vi "crop_input_images_float.vi"() -> ()   [LabVIEW 2011]
uses:
  global_vars.vi
  <vilib>/Utility/file.llb/Write To Spreadsheet File (I64).vi
panel:
  in  "dbl_gamma_correction":dbl=1.0
  in  "dbl_noise_threshold":dbl=20.0
  in  "update global variables":bool
  out "i32_First/last px":i32[][](graph)
  in  "safety margin":i32=5
  out "u8_ar_noise_mask":u8[][](array[numeric])
  out "input_line_plot 2":dbl[][](graph)
  in  "Tab Control":T1(tab)
  out "input_line_plot":dbl[][](graph)
  out "img_dist_input":T2(plugin-control)
  out "img_orig_input":T2(plugin-control)
  in  "i32_sel_input_image":i32
  in  "select row input":i32(slide) scale=0.0..1200.0
  in  "select row unwrapped":i32(slide) scale=0.0..1200.0
  out "img_dist_phaseMap":T2(plugin-control)
  out "img_orig_masked_with_dist":T2(plugin-control)
  out "noise_mask_line_plot":i32[](graph)
  in  "select row":i32(slide) scale=0.0..1200.0
  out "last px":i32
  out "first px":i32
  out "img_noise_mask":T2(plugin-control)
  in  "save data":bool
  out "i32_ar_displ_map":i32[][](array[numeric])
  out "crunching numbers":bool
  out "Intensity Graph":i32[][](graph)
  out "img_orig_unwrap":T2(plugin-control)
  in  "calc difference":bool
  out "Y Resolution":i32
  out "X Resolution":i32
  in  "update_cor":bool
  out "path_dist_files":path[](array[path])=[path "X:/Cloud Drives/Dropbox/Europhotonics/FringeMan/Image Storage/02_07/x-direction/dist/12_56_10-5.00fringes_0of4__capt_.png", path "X:/Cloud Drives/Dropbox/Europhotonics/FringeMan/Image Storage/02_07/x-direction/dist/12_56_10-5.00fringes_1of4__capt_.png", path "X:/Cloud Drives/Dropbox/Europhotonics/FringeMan/Image Storage/02_07/x-direction/dist/12_56_10-5.00fringes_2of4__capt_.png", path "X:/Cloud Drives/Dropbox/Europhotonics/FringeMan/Image Storage/02_07/x-direction/dist/12_56_10-5.00fringes_3of4__capt_.png"]
  out "path_orig_files":path[](array[path])=[path "X:/Cloud Drives/Dropbox/Europhotonics/FringeMan/Image Storage/02_07/x-direction/orig/12_56_10-5.00fringes_0of4__original_.png", path "X:/Cloud Drives/Dropbox/Europhotonics/FringeMan/Image Storage/02_07/x-direction/orig/12_56_10-5.00fringes_1of4__original_.png", path "X:/Cloud Drives/Dropbox/Europhotonics/FringeMan/Image Storage/02_07/x-direction/orig/12_56_10-5.00fringes_2of4__original_.png", path "X:/Cloud Drives/Dropbox/Europhotonics/FringeMan/Image Storage/02_07/x-direction/orig/12_56_10-5.00fringes_3of4__original_.png"]
  in  "dbl_ar_crop_correction":dbl[](array[numeric])=[0.0, 0.0, 0.0, 0.0] caption="crop_correction"
  in  "u8_y_center_cor":i16
  in  "u8_x_center_cor":i16=-20
  in  "radius correction":i16=-30
  out "img_dist_unwrap":T2(plugin-control)
  out "u8_ar_orig_phasemap":dbl[][](array[numeric])
  out "dbl_pxar_orig_unwrap":dbl[][](array[numeric])
  out "dbl_pxar_dist_unwrap":dbl[][](array[numeric])
  out "u8_pxar_orig":dbl[][][](array[numeric])
  in  "read orig":bool
  in  "read dist":bool
  out "u8_ar_dist_phasemap":dbl[][](array[numeric])
  in  "calculate \nphase map":bool
  out "u8_pxar_dist":dbl[][][](array[numeric])
  in  "Stop Button":bool
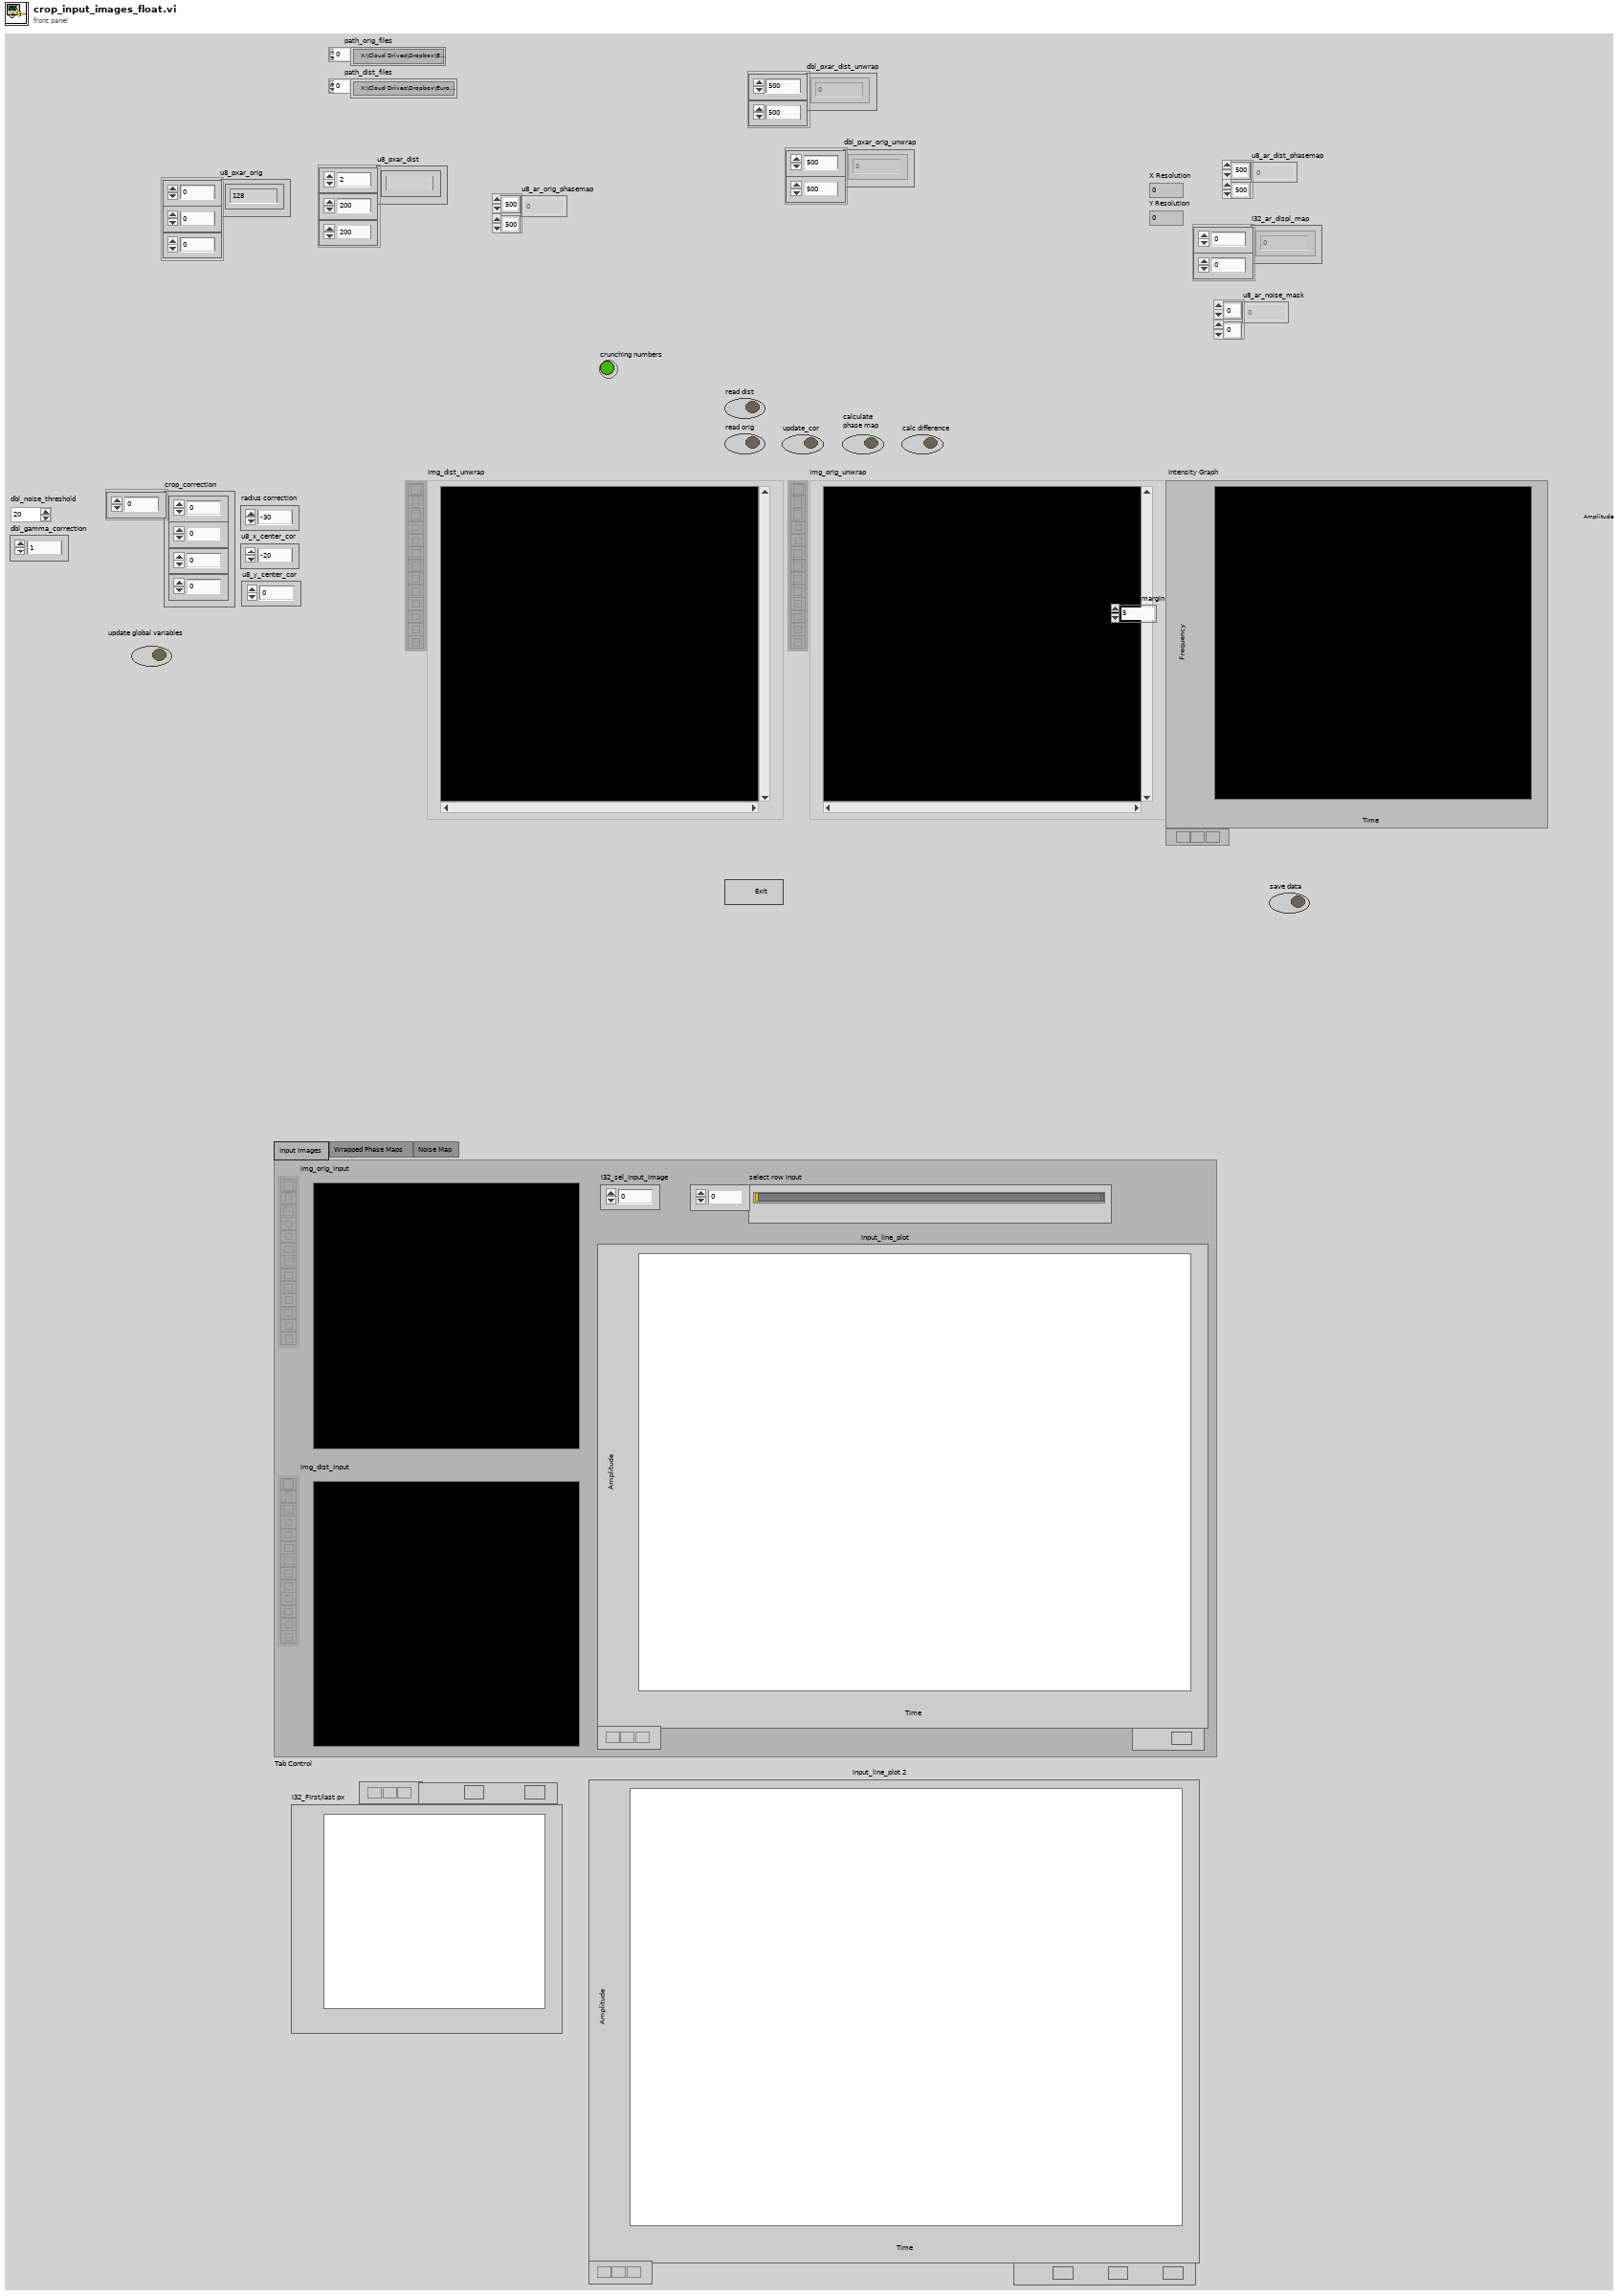
[diagram p1: front panel]
types:
  T1 = enum32{"Input Images", "Wrapped Phase Maps", "Noise Map"}
  T2 = typedef "IMAQ Image.ctl" = refnum<image>
  T3 = cluster{"radius correction":i16, "u8_x_center_cor":i16, "u8_y_center_cor":i16}
  T4 = typedef "Image Type" = u32
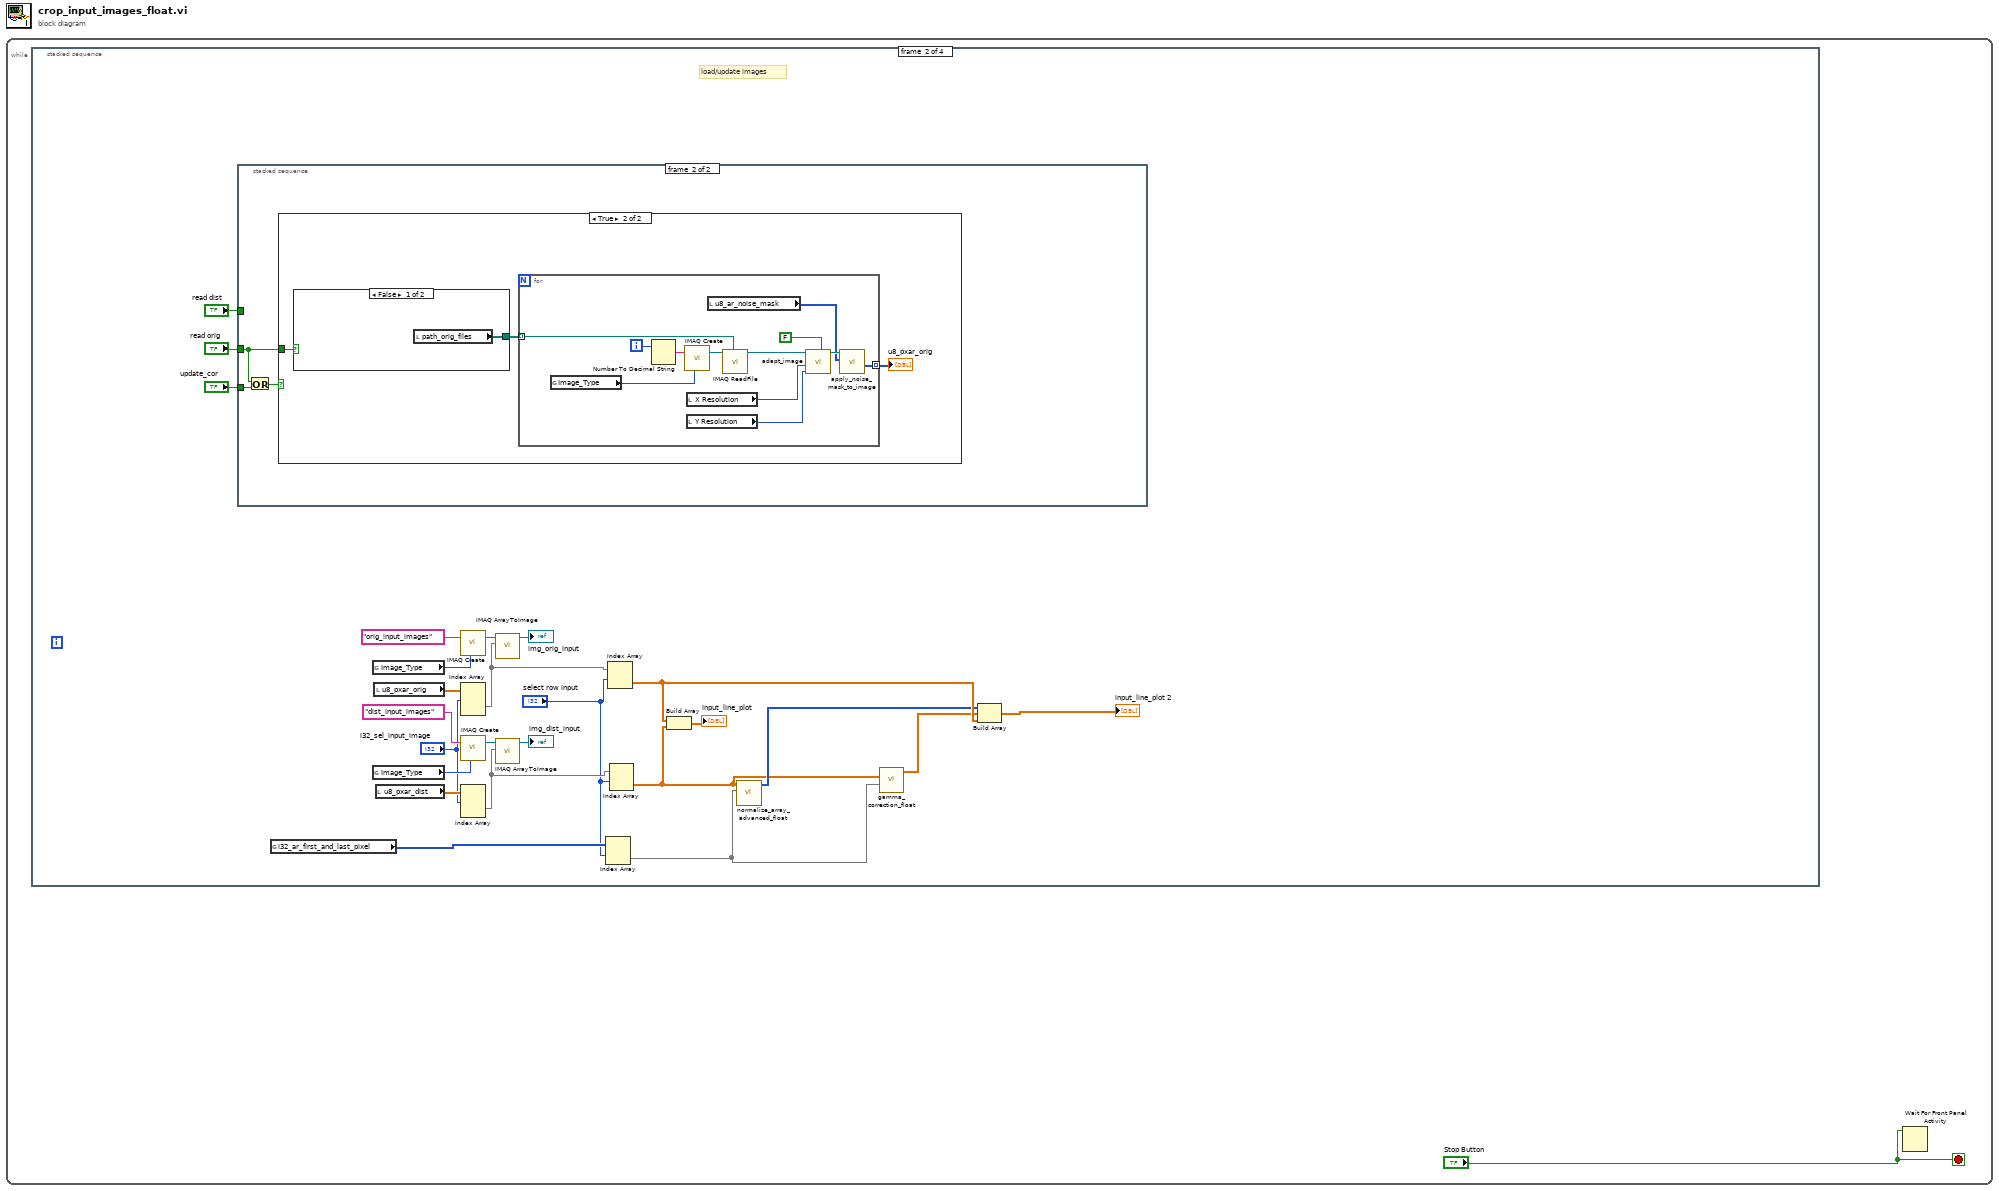
[diagram p0: block diagram]
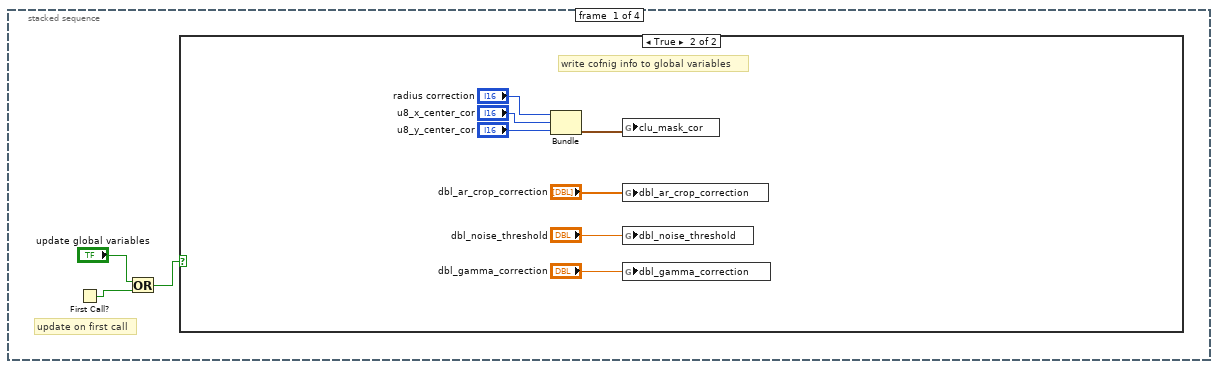
[diagram p2: hidden frame]
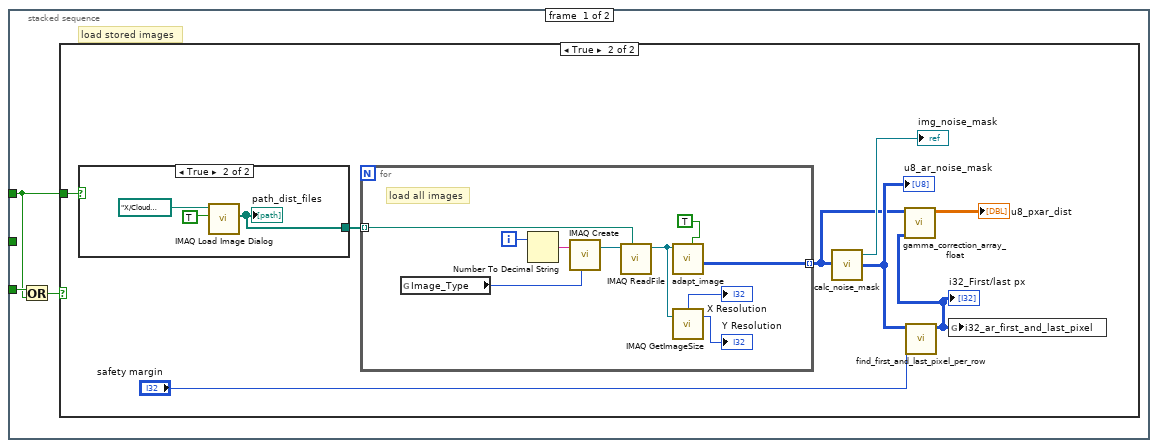
[diagram p4: hidden frame]
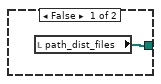
[diagram p6: hidden frame]
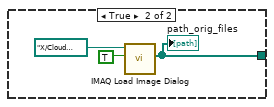
[diagram p8: hidden frame]
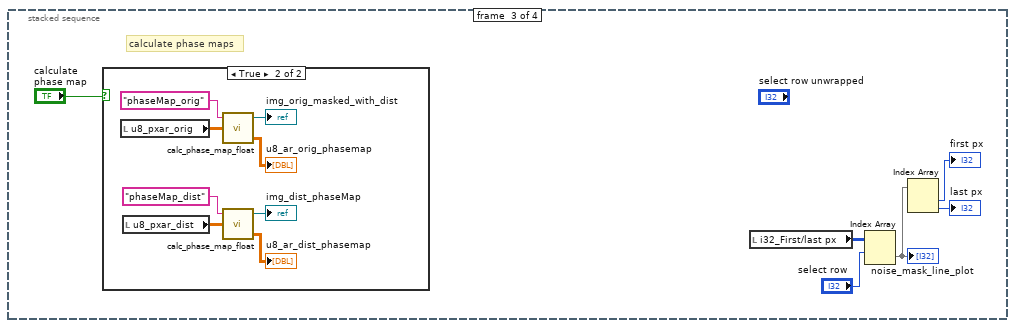
[diagram p9: hidden frame]
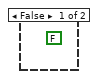
[diagram p10: hidden frame]
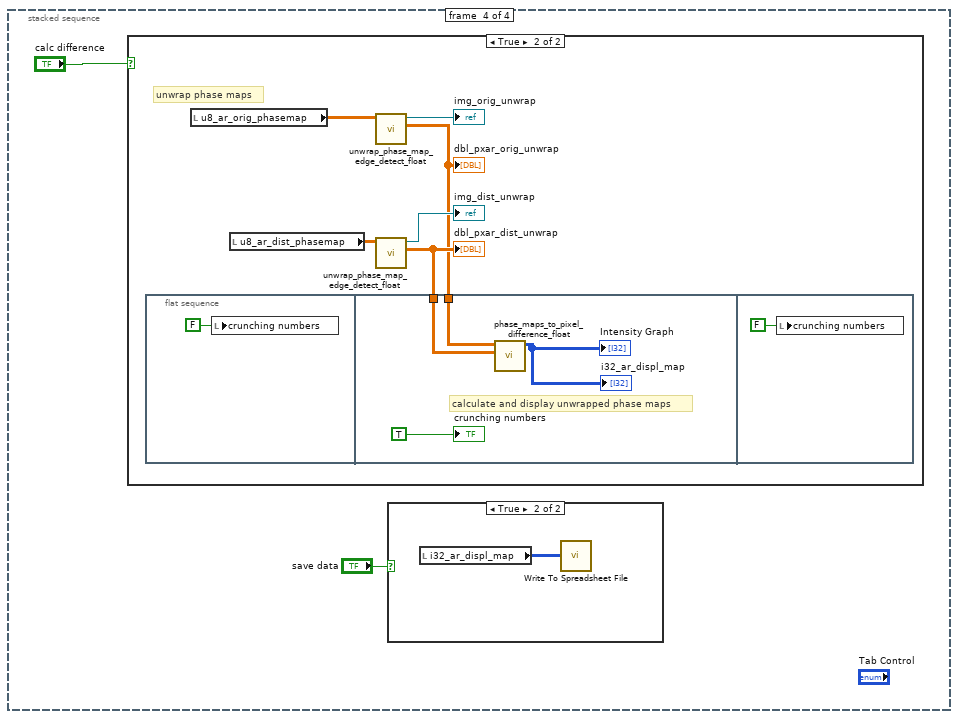
[diagram p11: hidden frame]
diagram:
  n1 = while {
    stop <- "Stop Button" stop-if-true
    n2 = stacked-sequence {
      frame #0 {
        # "update on first call"
        n3 = First Call?() -> (First Call?: T/F=w2:bool)
        n4 = Or(x="update global variables", y=w2) -> (x .or. y?=w3:bool)
        n5 = case shown="True" w3 {
          frame False {
          }
          frame True {
            # "write cofnig info to global variables"
            n6 = Bundle("radius correction"="radius correction", "u8_x_center_cor"="u8_x_center_cor", "u8_y_center_cor"="u8_y_center_cor") -> (w11:T3)  [unwired: 1 in]
            n7 = global write "global_vars.vi" "clu_mask_cor"(w11) -> ()
            n8 = global write "global_vars.vi" "dbl_ar_crop_correction"("dbl_ar_crop_correction") -> ()
            n9 = global write "global_vars.vi" "dbl_noise_threshold"("dbl_noise_threshold") -> ()
            n10 = global write "global_vars.vi" "dbl_gamma_correction"("dbl_gamma_correction") -> ()
          }
        }
      }
      frame #1 {
        # "load/update images"
        n11 = stacked-sequence {
          tunnel: "update_cor" -> [w39 w63]
          tunnel: "read dist" -> [w37 _]
          tunnel: "read orig" -> [_ w62]
          frame #0 {
            # "load stored images"
            n12 = Or(x=w39, y=w37) -> (x .or. y?=w38:bool)
            n13 = case shown="True" w38 {
              tunnel: w37 -> [_ w46]
              frame False {
              }
              frame True {
                n14 = case shown="True" w46 {
                  tunnel: [w48 w51] -> w47
                  frame False {
                    n15 = local read "path_dist_files"() -> (w48:path[])
                  }
                  frame True {
                    n16 = call "IMAQ Load Image Dialog"("Multiple Files? (No)"=TRUE, "Start Path"=path "X:/Cloud Drives/Dropbox/Europhotonics/FringeMan/Image Storage") -> ("Paths"=w51:path[])  [unwired: 7 in, 2 out]
                    "path_dist_files" <- w51
                  }
                }
                n17 = for {
                  tunnel: w47 -> [w57] mode=indexing
                  tunnel: [w53] -> w42 mode=indexing
                  i -> [w61]
                  # "load all images"
                  n18 = global read "global_vars.vi" "Image_Type"() -> (w58:T4)
                  n19 = Number To Decimal String(number=w61) -> (decimal integer string=w60:string)  [unwired: 1 in]
                  n20 = call "IMAQ Create"("Image Name"=w60, "Image Type"=w58) -> ("New Image"=w59:T2)  [unwired: 2 in, 2 out]
                  n21 = call "IMAQ ReadFile"("File Path"=w57, "Image"=w59) -> ("Image Out"=w54:T2)  [unwired: 5 in, 4 out]
                  n22 = call "adapt_image.vi"("captured image?"=TRUE, "orig_imageIn"=w54) -> ("adapted image px array"=w53:u8[][])  [unwired: 7 in, 2 out]
                  n23 = call "IMAQ GetImageSize"("Image"=w54) -> ("Y Resolution"=→"Y Resolution":i32, "X Resolution"=→"X Resolution":i32)  [unwired: 3 in, 1 out]
                }
                n24 = call "calc_noise_mask.vi"("u8_ar_image_pixel_array"=w42) -> ("u8_ar_noise_mask"=w43:u8[][], "img_noise mask"=→"img_noise_mask":T2)  [unwired: 3 in]
                "u8_ar_noise_mask" <- w43
                n25 = call "find_first_and_last_pixel_per_row.vi"("safety margin"="safety margin", "u8_ar_mask"=w43) -> ("i32_ar_first_and_last_pixel"=w40:i32[][])  [unwired: 9 in]
                "i32_First/last px" <- w40
                n26 = call "gamma_correction_array_float.vi"("i32_ar_first_and_last_pixel"=w40, "adapted image px array"=w42) -> ("i16_normalized unwrapped array"=→"u8_pxar_dist":dbl[][][])  [unwired: 9 in]
                n27 = global write "global_vars.vi" "i32_ar_first_and_last_pixel"(w40) -> ()
              }
            }
          }
          frame #1 {
            n28 = Or(x=w62, y=w63) -> (x .or. y?=w64:bool)
            n29 = case shown="True" w64 {
              tunnel: w62 -> [_ w66]
              frame False {
              }
              frame True {
                n30 = case shown="False" w66 {
                  tunnel: [w68 w70] -> w67
                  frame False {
                    n31 = local read "path_orig_files"() -> (w68:path[])
                  }
                  frame True {
                    n32 = call "IMAQ Load Image Dialog"("Multiple Files? (No)"=TRUE, "Start Path"=path "X:/Cloud Drives/Dropbox/Europhotonics/FringeMan/Image Storage") -> ("Paths"=w70:path[])  [unwired: 7 in, 2 out]
                    "path_orig_files" <- w70
                  }
                }
                n33 = for {
                  tunnel: w67 -> [w83] mode=indexing
                  tunnel: [w73] -> w65 mode=indexing
                  i -> [w79]
                  n34 = global read "global_vars.vi" "Image_Type"() -> (w80:T4)
                  n35 = Number To Decimal String(number=w79) -> (decimal integer string=w82:string)  [unwired: 1 in]
                  n36 = call "IMAQ Create"("Image Name"=w82, "Image Type"=w80) -> ("New Image"=w81:T2)  [unwired: 2 in, 2 out]
                  n37 = local read "X Resolution"() -> (w77:i32)
                  n38 = local read "Y Resolution"() -> (w76:i32)
                  n39 = local read "u8_ar_noise_mask"() -> (w72:u8[][])
                  n40 = call "IMAQ ReadFile"("File Path"=w83, "Image"=w81) -> ("Image Out"=w78:T2)  [unwired: 5 in, 4 out]
                  n41 = call "adapt_image.vi"("captured image?"=FALSE, "captImage_Y_Resolution"=w76, "captImage_X_Resolution"=w77, "orig_imageIn"=w78) -> ("adapted image"=w74:T2)  [unwired: 5 in, 2 out]
                  n42 = call "apply_noise_mask_to_image.vi"("u8_ar_noise_mask in"=w72, "Refnum in"=w74) -> ("Image Pixels (U8)"=w73:u8[][])  [unwired: 7 in, 2 out]
                }
                "u8_pxar_orig" <- w65
              }
            }
          }
        }
        n43 = global read "global_vars.vi" "i32_ar_first_and_last_pixel"() -> (w19:i32[][])
        n44 = global read "global_vars.vi" "Image_Type"() -> (w31:T4)
        n45 = global read "global_vars.vi" "Image_Type"() -> (w28:T4)
        n46 = local read "u8_pxar_orig"() -> (w32:dbl[][][])
        n47 = local read "u8_pxar_dist"() -> (w33:dbl[][][])
        n48 = call "IMAQ Create"("Image Name"="orig_input_images", "Image Type"=w31) -> ("New Image"=w26:T2)  [unwired: 2 in, 2 out]
        n49 = Index Array(array=w32, index (dim 0)="i32_sel_input_image") -> (element=w23:dbl[][])  [unwired: 2 in]
        n50 = call "IMAQ Create"("Image Name"="dist_input_images", "Image Type"=w28) -> ("New Image"=w27:T2)  [unwired: 2 in, 2 out]
        n51 = Index Array(array=w33, index (dim 0)="i32_sel_input_image") -> (element=w22:dbl[][])  [unwired: 2 in]
        n52 = call "IMAQ ArrayToImage"("Image Pixels (U8)"=w23, "Image"=w26) -> ("Image Out"=→"img_orig_input":T2)  [unwired: 8 in, 1 out]
        n53 = call "IMAQ ArrayToImage"("Image Pixels (U8)"=w22, "Image"=w27) -> ("Image Out"=→"img_dist_input":T2)  [unwired: 8 in, 1 out]
        n54 = Index Array(array=w19, index (row)="select row input") -> (element=w14:i32[])  [unwired: 1 in]
        n55 = Index Array(array=w23, index (row)="select row input") -> (element=w20:dbl[])  [unwired: 1 in]
        n56 = Index Array(array=w22, index (row)="select row input") -> (element=w12:dbl[])  [unwired: 1 in]
        n57 = Build Array(w20, w12) -> (→"input_line_plot":dbl[][])
        n58 = call "normalize_array_advanced_float.vi"("i32_ar_first_and_last_pixel"=w14, "unwrapped array"=w12) -> ("normalized unwrapped array"=w17:u8[])  [unwired: 5 in, 4 out]
        n59 = call "gamma_correction_float.vi"("i32_ar_first_and_last_pixel"=w14, "u8_pxar_dist"=w12) -> ("i16_normalized unwrapped array"=w13:dbl[])  [unwired: 9 in]
        n60 = Build Array(w17, w13, w20) -> (→"input_line_plot 2":dbl[][])
      }
      frame #2 {
        # "calculate phase maps"
        n61 = case shown="True" "calculate \nphase map" {
          frame False {
            (unwired) FALSE
          }
          frame True {
            n62 = local read "u8_pxar_orig"() -> (w92:dbl[][][])
            n63 = local read "u8_pxar_dist"() -> (w96:dbl[][][])
            n64 = call "calc_phase_map_float.vi"("u8_ar_image_pixel_array"=w92, "image name"="phaseMap_orig" ("String")) -> ("raw phase map array"=→"u8_ar_orig_phasemap":dbl[][], "phase map"=→"img_orig_masked_with_dist":T2)  [unwired: 2 in]
            n65 = call "calc_phase_map_float.vi"("u8_ar_image_pixel_array"=w96, "image name"="phaseMap_dist" ("String")) -> ("raw phase map array"=→"u8_ar_dist_phasemap":dbl[][], "phase map"=→"img_dist_phaseMap":T2)  [unwired: 2 in]
          }
        }
        n66 = local read "i32_First/last px"() -> (w87:i32[][])
        n67 = Index Array(array=w87, index (row)="select row") -> (element=w84:i32[])  [unwired: 1 in]
        "noise_mask_line_plot" <- w84
        n68 = Index Array(array=w84) -> (element #1=→"first px":i32, element #2=→"last px":i32)  [unwired: 2 in]
      }
      frame #3 {
        n69 = case shown="True" "calc difference" {
          frame False {
          }
          frame True {
            # "unwrap phase maps"
            n70 = flat-sequence {
              tunnel: w103 -> [w108]
              tunnel: w102 -> [w109]
              frame #0 {
                n71 = local write "crunching numbers"(FALSE) -> ()
              }
              frame #1 {
                # "calculate and display unwrapped phase maps"
                n72 = call "phase_maps_to_pixel_difference_float.vi"("dist phase map"=w108, "oirg phase map"=w109) -> ("displacement map"=→"Intensity Graph" →"i32_ar_displ_map":i32[][])  [unwired: 9 in]
                "crunching numbers" <- TRUE
              }
              frame #2 {
                n73 = local write "crunching numbers"(FALSE) -> ()
              }
            }
            n74 = local read "u8_ar_orig_phasemap"() -> (w101:dbl[][])
            n75 = local read "u8_ar_dist_phasemap"() -> (w104:dbl[][])
            n76 = call "unwrap_phase_map_edge_detect_float.vi"("u8_ar_dist_phasemap"=w101) -> ("df_ar_unwrapped_px_ar"=w102:dbl[][], "Refnum out"=→"img_orig_unwrap":T2)  [unwired: 9 in]
            "dbl_pxar_orig_unwrap" <- w102
            n77 = call "unwrap_phase_map_edge_detect_float.vi"("u8_ar_dist_phasemap"=w104) -> ("df_ar_unwrapped_px_ar"=w103:dbl[][], "Refnum out"=→"img_dist_unwrap":T2)  [unwired: 9 in]
            "dbl_pxar_dist_unwrap" <- w103
          }
        }
        n78 = case shown="True" "save data" {
          frame False {
          }
          frame True {
            n79 = local read "i32_ar_displ_map"() -> (w100:i32[][])
            n80 = call-poly <vilib>:"Write To Spreadsheet File.vi"("2D data"=w100) -> ()  [unwired: 7 in, 1 out]
          }
        }
      }
    }
    n81 = Wait For Front Panel Activity(3:"Stop Button") -> ()  [unwired: 2 in, 1 out]
  }
